vi "SetFreq.vi"(6 "Reference Frequency (Hz)":dbl, 7 "Enable Reference Frequency":bool, 8 "error in (no error)":errorcluster, 9 "Offset Frequency (Hz)":dbl, 10 "Frequency (Hz)":dbl=100000.0, 11 "SigGen_MXG in":refnum<class "SigGen_MXG.lvclass">) -> (0 "error out":errorcluster, 3 "SigGen_MXG out":refnum<class "SigGen_MXG.lvclass">)   [LabVIEW 2014, in "SigGen_MXG.lvclass"]
uses:
  SigGen_MXG.lvclass
  SigGen_MXG.lvclass/SigGen_MXG.ctl
  data/Agilent PSG MXG Series.lvlib
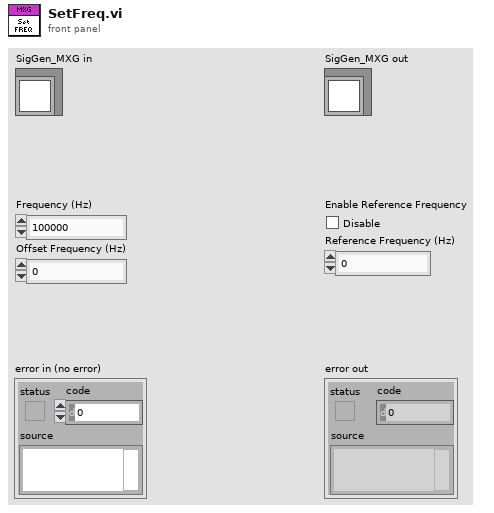
[diagram p1: front panel]
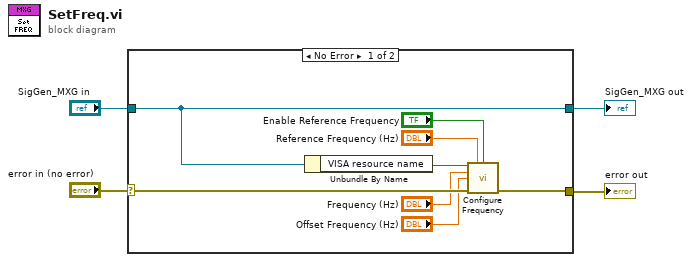
[diagram p0: block diagram]
diagram:
  n1 = case shown="No Error" "error in (no error)" {
    selector: "error in (no error)" -> [w12 w14]
    tunnel: [w11 w14] -> w3
    tunnel: [w10 w13] -> w1
    tunnel: "SigGen_MXG in" -> [w10 w13]
    frame No Error {
      n2 = Unbundle By Name(w10) -> ("VISA resource name"=w9:refnum<visa-resource-name>)
      n3 = call "Configure Frequency.vi"("VISA resource name"=w9, "Reference Frequency (0 Hz)"="Reference Frequency (Hz)", "Enable Reference Frequency (F:Disable)"="Enable Reference Frequency", "Frequency (100 kHz)"="Frequency (Hz)", "Offset Frequency (0 Hz)"="Offset Frequency (Hz)", "error in (no error)"=w12) -> ("error out"=w11:errorcluster)  [unwired: 3 in, 6 out]
    }
    frame Error {
    }
  }
  "error out" <- w3
  "SigGen_MXG out" <- w1
